vi "Open VI Panel.vi"(8 "error in":errorcluster, 11 "VI":refnum<vi>) -> (0 "error out":errorcluster)   [LabVIEW 2022 SP3, in "HW-210-manager.lvlib"]
doc: "Open and activate the panel of the specified VI.\n_____\nBased on DQMH Project Template 7.0.1.1316."
uses:
  HW-210-manager.lvlib
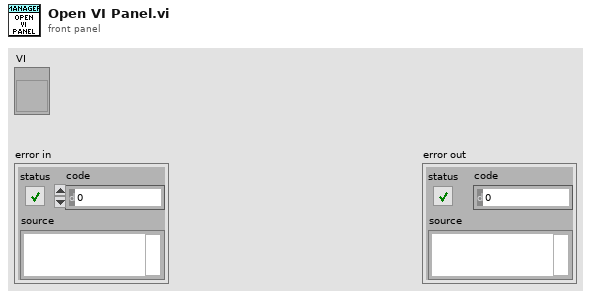
[diagram p1: front panel]
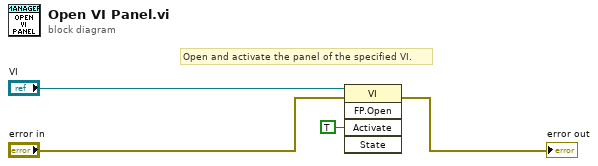
[diagram p0: block diagram]
diagram:
  # "Open and activate the panel of the specified VI."
  n1 = invoke class="VI" method="FP.Open"(reference="VI", error in="error in", "Activate"=TRUE ("Activate?")) -> (error out=→"error out":errorcluster)  [unwired: 2 in, 4 out]
